vi "NiFPGA Write FIFO - Boolean.vi"(6 "Timeout":u32, 8 "error in (no error)":errorcluster, 9 "Data":bool[](array[boolean]), 10 "FIFO":u32, 11 "Session":u32) -> (0 "error out":errorcluster, 3 "Session Out":u32, 4 "Empty Elements Remaining":u32)   [LabVIEW 2010, in "FPGA Interface Wrapper.lvlib"]
doc: "Writes to a FIFO of booleans."
uses:
  <userlib>/_FPGA Interface Advanced Tools/FPGA Interface Wrapper/FPGA Interface Wrapper.lvlib
  NiFpga.dll
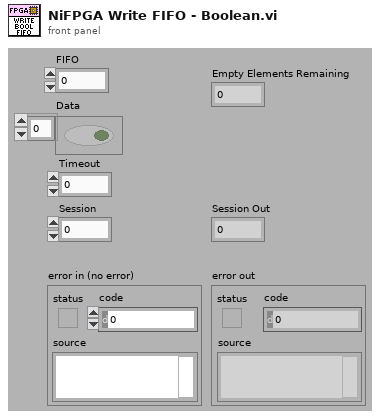
[diagram p1: front panel]
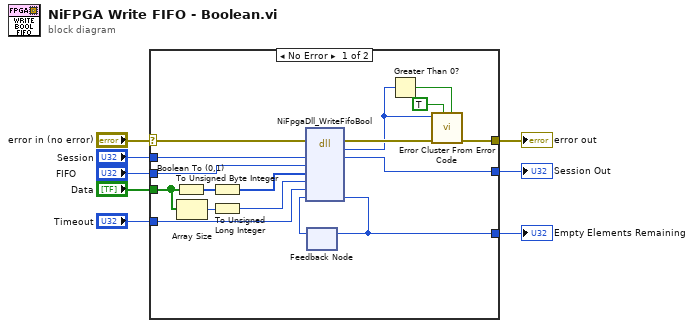
[diagram p0: block diagram]
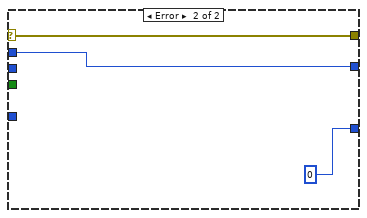
[diagram p2: hidden frame]
diagram:
  n1 = case shown="No Error" "error in (no error)" {
    selector: "error in (no error)" -> [w25 w27]
    tunnel: [w12 w27] -> w7
    tunnel: "Session" -> [w24 w28]
    tunnel: [w23 w28] -> w5
    tunnel: "FIFO" -> [w22 _]
    tunnel: "Timeout" -> [w21 _]
    tunnel: [w9 u64 0 ("Elements Remaining")] -> w2
    tunnel: "Data" -> [w17 _]
    frame No Error {
      n2 = Boolean To (0,1)(Boolean=w17) -> (0, 1=w20:i16[])
      n3 = Array Size(array=w17) -> (size(s)=w18:i32)
      n4 = To Unsigned Byte Integer(number=w20) -> (unsigned 8bit integer=w19:u8[])
      n5 = To Unsigned Long Integer(number=w18) -> (unsigned 32bit integer=w16:u32)
      n6 = feedback #1() -> (w10:u64)  [unwired: 1 in]
      n7 = dll-call lib="NiFpga.dll" fn="NiFpgaDll_WriteFifoBool"(error in=w25, "Session"=w24, "FIFO"=w22, "Data"=w19, "Number of Elements"=w16, "Timeout"=w21, "Empty Elements Remaining"=w10) -> (error out=w13:errorcluster, "Status"=w11:i32, "Session"=w23:u32, "Empty Elements Remaining"=w9:u64)  [unwired: 6 in, 1 out]
      n8 = feedback-in #1(w9) -> ()
      n9 = Greater Than 0?(x=w11) -> (x > 0?=w14:bool)
      n10 = call <vilib>:"Error Cluster From Error Code.vi"("is warning? (False)"=w14, "show call chain? (False)"=TRUE, "error in (no error)"=w13, "error code (0)"=w11) -> ("error out"=w12:errorcluster)  [unwired: 5 in]
    }
    frame Error {
    }
  }
  "error out" <- w7
  "Session Out" <- w5
  "Empty Elements Remaining" <- w2
